vi "SP Unwrap Phase.vi"(0 "Phase":dbl[](array[numeric])) -> (1 "Unwrapped Phase":dbl[](array[numeric]), 2 "error":i32)   [LabVIEW 2011]
doc: "Unwraps the <B>Phase</B> array by eliminating discontinuities whose absolute values exceed pi."
uses:
  Program Files/National Instruments/LabVIEW 2011/resource/lvanlys.dll
panel:
  # "Unwrap Phase"
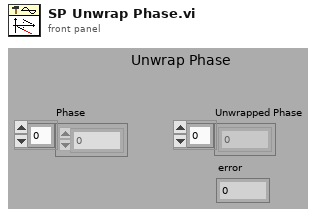
[diagram p1: front panel]
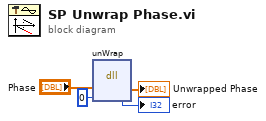
[diagram p0: block diagram]
diagram:
  n1 = dll-call lib="C:/Program Files/National Instruments/LabVIEW 2011/resource/lvanlys.*" fn="unWrap"("Phase"="Phase", "error"=0) -> ("Phase"=→"Unwrapped Phase":dbl[], "error"=→"error":i32)  [unwired: 3 in, 3 out]
